vi "Build Xfer Matrix.vi"(7 "NumBins":i32, 8 "error in (no error)":errorcluster, 10 "Voltage":dbl[](array[numeric]), 11 "DMA in":refnum<class "DMA.lvclass">) -> (0 "error out":errorcluster, 2 "xfer":dbl[][](array[numeric]), 3 "DMA out":refnum<class "DMA.lvclass">)   [LabVIEW 2015, in "DMA.lvclass"]
uses:
  DMA.lvclass
  DMA.lvclass/DMA.ctl
  Particle Class/Particle Properties.lvclass/Particle Properties.ctl
  Accessors/Read Particle.vi
  Accessors/Read ri.vi
  Accessors/Read ro.vi
  Accessors/Read Leff.vi
  Accessors/Read Qex.vi
  Accessors/Read Qsh.vi
  Particle Class/Accessors/Write D.vi
  Particle Class/Accessors/Write # of charges.vi
  Particle Class/Calculate Charging Efficiency.vi
  Particle Class/Particle Properties.lvclass
panel:
  out "XY Graph":cluster{dbl[], dbl[]}(graph)
  out "Array 4":dbl[](array[numeric])
  out "kappa":dbl[][][](array[numeric])
  out "Array 2":dbl[][][](array[numeric])
  out "Array":dbl[][][](array[numeric])
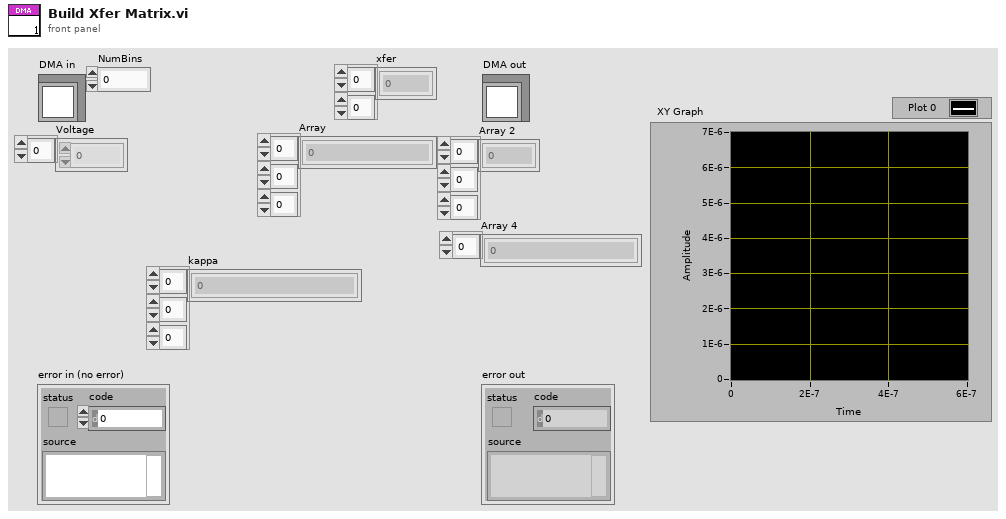
[diagram p1: front panel]
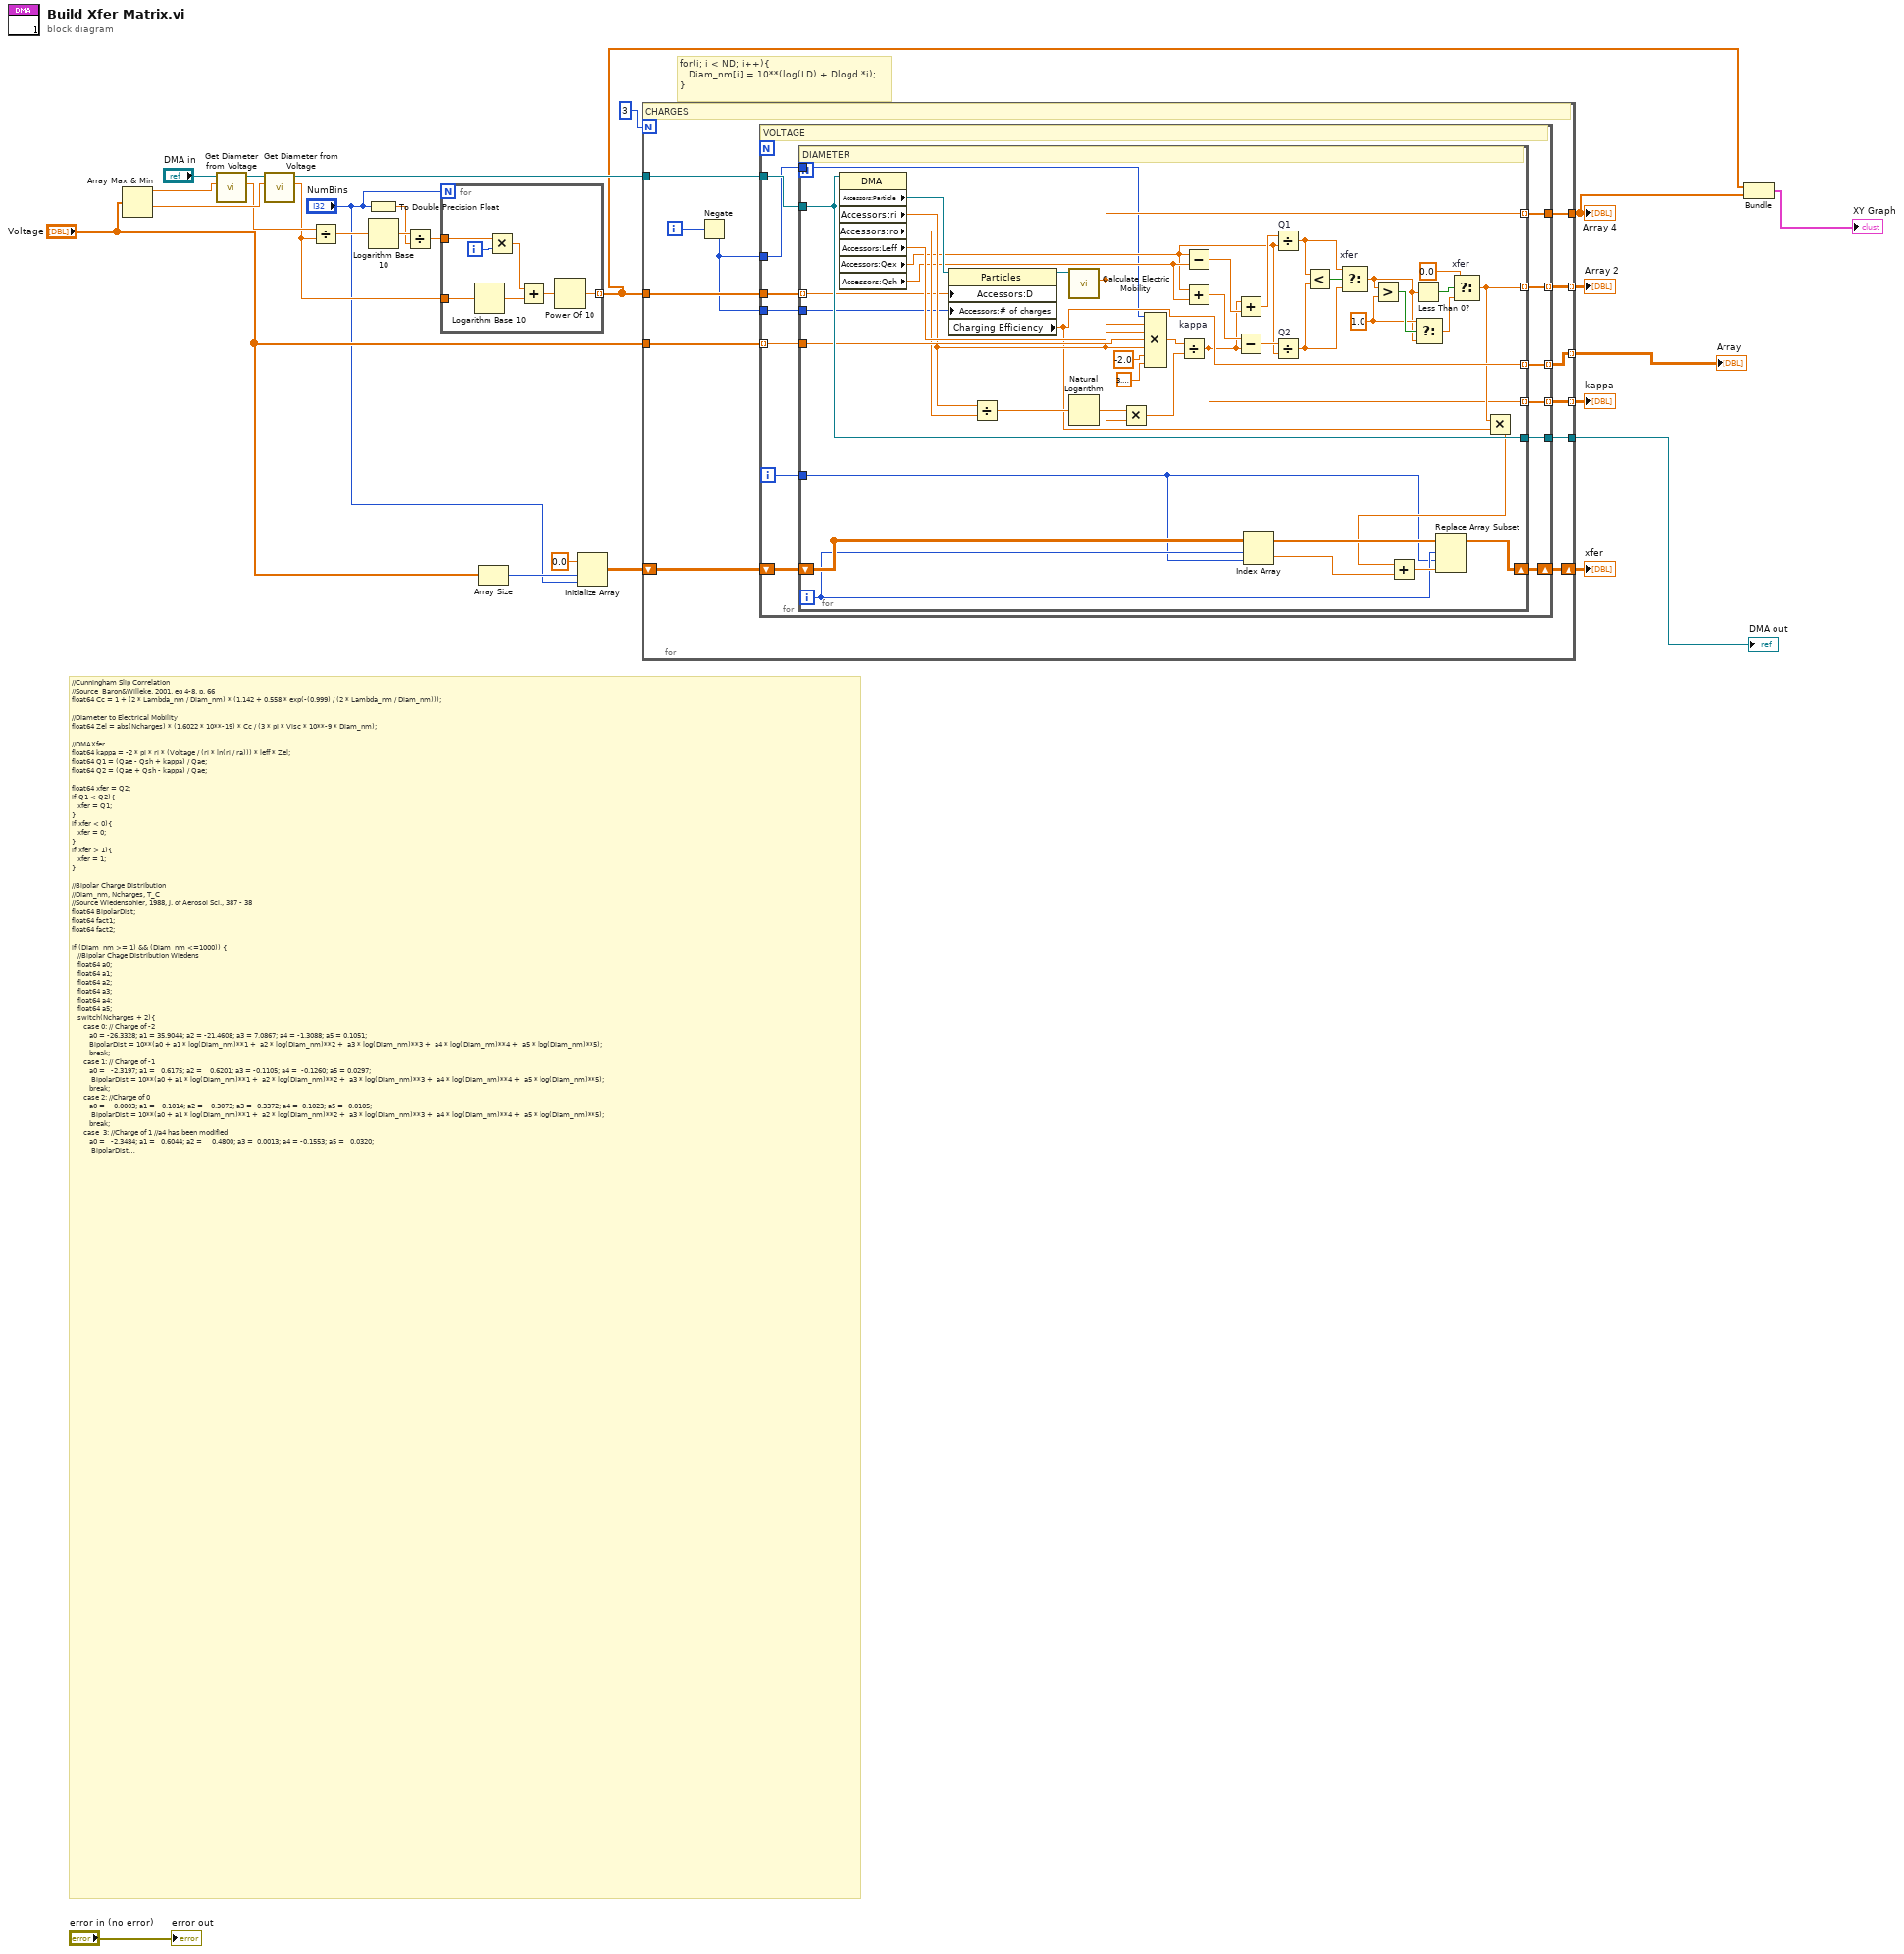
[diagram p0: block diagram]
diagram:
  # "for(i; i < ND; i++){\n   Diam_nm[i] = 10**(log(LD) + Dlogd *i);\n}"
  # "//Cunningham Slip Correlation\n//Source  Baron&Willeke, 2001, eq 4-8, p. 66\nfloat64 Cc = 1 + (2 * Lambda_nm / Diam_nm) * (1.142 + 0.558 * exp(-(0.999) / (2 * Lambda_nm / Diam_nm)));\n\n//Diameter to Electrical Mobility\nfloat64 Zel = abs(Ncharges) * (1.6022 * 10**-19) * Cc / (3 * pi * Visc * 10**-9 * Diam_nm);\n\n//DMAXfer\nfloat64 kappa = -2 * pi * ri * (Voltage / (ri * ln(ri / ra))) * leff * Zel;\nfloat64 Q1 = (Qae - Qsh + kappa) / Qae;\nfloat64 Q2 = (Qae + Qsh - kappa) / Qae;\n\nfloat64 xfer = Q2;\nif(Q1 < Q2){\n   xfer = Q1;\n}\nif(xfer < 0){\n   xfer = 0;\n}\nif(xfer > 1){\n   xfer = 1;\n}\n\n//Bipolar Charge Distribution\n//Diam_nm, Ncharges, T_C\n//Source Wiedensohler, 1988, J. of Aerosol Sci., 387 - 38\nfloat64 BipolarDist;\nfloat64 fact1;\nfloat64 fact2;\n\nif((Diam_nm >= 1) && (Diam_nm <=1000)) {\n   //Bipolar Chage Distribution Wiedens\n   float64 a0;\n   float64 a1;\n   float64 a2;\n   float64 a3;\n   float64 a4;\n   float64 a5;\n   switch(Ncharges + 2){\n      case 0: // Charge of -2\n         a0 = -26.3328; a1 = 35.9044; a2 = -21.4608; a3 = 7.0867; a4 = -1.3088; a5 = 0.1051;\n         BipolarDist = 10**(a0 + a1 * log(Diam_nm)**1 +  a2 * log(Diam_nm)**2 +  a3 * log(Diam_nm)**3 +  a4 * log(Diam_nm)**4 +  a5 * log(Diam_nm)**5);\n         break;\n      case 1: // Charge of -1\n         a0 =   -2.3197; a1 =   0.6175; a2 =    0.6201; a3 = -0.1105; a4 =  -0.1260; a5 = 0.0297;\n          BipolarDist = 10**(a0 + a1 * log(Diam_nm)**1 +  a2 * log(Diam_nm)**2 +  a3 * log(Diam_nm)**3 +  a4 * log(Diam_nm)**4 +  a5 * log(Diam_nm)**5);\n         break;\n      case 2: //Charge of 0\n         a0 =   -0.0003; a1 =  -0.1014; a2 =    0.3073; a3 = -0.3372; a4 =  0.1023; a5 = -0.0105;\n          BipolarDist = 10**(a0 + a1 * log(Diam_nm)**1 +  a2 * log(Diam_nm)**2 +  a3 * log(Diam_nm)**3 +  a4 * log(Diam_nm)**4 +  a5 * log(Diam_nm)**5);\n         break;\n      case  3: //Charge of 1 //a4 has been modified\n         a0 =   -2.3484; a1 =   0.6044; a2 =     0.4800; a3 =  0.0013; a4 = -0.1553; a5 =   0.0320;\n          BipolarDist = 10**(a0 + a1 * log(Diam_nm)**1 +  a2 * log(Diam_nm)**2 +  a3 * log(Diam_nm)**3 +  a4 * log(Diam_nm)**4 +  a5 * log(Diam_nm)**5);\n         break;\n      case  4: //Charge of 2 //a5 has been modified\n         a0 = -44.4756; a1 = 79.3772; a2 =  -62.8900; a3 = 26.4492; a4 = -5.7480; a5 =  0.5049;\n         BipolarDist = 10**(a0 + a1 * log(Diam_nm)**1 +  a2 * log(Diam_nm)**2 +  a3 * log(Diam_nm)**3 +  a4 * log(Diam_nm)**4 +  a5 * log(Diam_nm)**5);\n         break;\n      default:\n         //Bipolar Chage Distribution Gunn\n         fact1 = (1.6022*10**-19) / sqrt(4 * pi**2 * (8.8542*10**-12) * Diam_nm  * 10**-9 * (1.3807*10**-23) * T_K);\n         fact2 = 2 * pi * (8.8542*10**-12) * Diam_nm * 10**-9 * (1.3807*10**-23) * T_K / (1.6022*10**-19) /  (1.6022*10**-19);\n         BipolarDist = fact1 * exp(-1 * (Ncharges - fact2 * ln(1 * 0.875))**2 / 2 / fact2);\n         break;\n   }\n}\nelse {\n   if((Diam_nm > 1000) && (Diam_nm <= 2000)) {\n      //Bipolar Chage Distribution Gunn\n      fact1 = (1.6022*10**-19) / sqrt(4 * pi**2 * (8.8542*10**-12) * Diam_nm  * 10**-9 * (1.3807*10**-23) * T_K);\n      fact2 = 2 * pi * (8.8542*10**-12) * Diam_nm * 10**-9 * (1.3807*10**-23) * T_K / (1.6022*10**-19) /  (1.6022*10**-19);\n      BipolarDist = fact1 * exp(-1 * (Ncharges - fact2 * ln(1 * 0.875))**2 / 2 / fact2);\n   }\n   else{\n      //Return NaN\n      BipolarDist = NaN;\n   }\n}\n\n Output = xfer * BipolarDist;"
  n1 = Array Max & Min(array="Voltage") -> (max value=w24:dbl, min value=w21:dbl)  [unwired: 2 out]
  n2 = call "Get Diameter from Voltage.vi"("Vin"=w24, "DMA in"="DMA in") -> ("Dout"=w19:dbl, "DMA out"=w22:refnum<class "DMA.lvclass">)  [unwired: 7 in, 1 out]
  n3 = call "Get Diameter from Voltage.vi"("Vin"=w21, "DMA in"=w22) -> ("Dout"=w14:dbl, "DMA out"=w20:refnum<class "DMA.lvclass">)  [unwired: 7 in, 1 out]
  n4 = Divide(x=w19, y=w14) -> (x/y=w18:dbl)
  n5 = To Double Precision Float(number="NumBins") -> (double precision float=w16:dbl)
  n6 = Logarithm Base 10(1:w18) -> (0:w17:dbl)
  n7 = Divide(x=w17, y=w16) -> (x/y=w15:dbl)
  n8 = for {
    N: "NumBins" -> [_]
    tunnel: w15 -> [w30]
    tunnel: w14 -> [w33]
    tunnel: [w27] -> w2 mode=indexing
    i -> [w31]
    n9 = Logarithm Base 10(1:w33) -> (0:w32:dbl)
    n10 = Multiply(x=w30, y=w31) -> (x*y=w29:dbl)
    n11 = Add(x=w29, y=w32) -> (x+y=w28:dbl)
    n12 = Power Of 10(x=w28) -> (10^x=w27:dbl)
  }
  n13 = Array Size(array="Voltage") -> (size(s)=w11:i32)
  n14 = Initialize Array(0.0 ("element"), w11, "NumBins") -> (w10:dbl[][])
  n15 = for {
    N: 3 -> [_]
    tunnel: [w45] -> w25
    tunnel: "Voltage" -> [w44]
    tunnel: w20 -> [w43]
    tunnel: w2 -> [w42]
    shift-right: [w40] -> w7
    shift-left: w10 -> [w41]
    tunnel: [w39] -> w6 mode=indexing
    tunnel: [w38] -> w5 mode=indexing
    tunnel: [w37] -> w4 mode=indexing
    tunnel: [w36] -> w3
    i -> [w35]
    # "CHARGES"
    n16 = Negate(x=w35) -> (-x=w34:i32)
    n17 = for {
      tunnel: [w58] -> w45
      tunnel: w44 -> [w57] mode=indexing
      tunnel: w43 -> [w56]
      tunnel: w42 -> [w55]
      tunnel: w34 -> [w54]
      shift-right: [w52] -> w40
      shift-left: w41 -> [w53]
      tunnel: [w50] -> w39 mode=indexing
      tunnel: [w49] -> w38 mode=indexing
      tunnel: [w48] -> w37 mode=indexing
      tunnel: [w47] -> w36
      tunnel: w34 -> [w46]
      i -> [w51]
      # "VOLTAGE"
      n18 = for {
        tunnel: w56 -> [w100]
        tunnel: w57 -> [w95]
        tunnel: [w100] -> w58
        tunnel: w55 -> [w73] mode=indexing
        tunnel: w54 -> [w61]
        shift-right: [w69] -> w52
        shift-left: w53 -> [w70]
        tunnel: w51 -> [w66]
        tunnel: [w64] -> w50 mode=indexing
        tunnel: [w63] -> w49 mode=indexing
        tunnel: [w62] -> w48 mode=indexing
        tunnel: [w60] -> w47 mode=indexing
        tunnel: w46 -> [w59]
        i -> [w67]
        w76 = 1.0 ("y")
        # "DIAMETER"
        n19 = property class="DMA"(reference=w100) -> ("Accessors:Particle"=w99:refnum<class "Particle Properties.lvclass">, "Accessors:ri"=w90:dbl, "Accessors:ro"=w93:dbl, "Accessors:Leff"=w94:dbl, "Accessors:Qex"=w82:dbl, "Accessors:Qsh"=w86:dbl)  [unwired: 1 in, 2 out]
        n20 = property class="Particles"(reference=w99, "Accessors:D"=w73, "Accessors:# of charges"=w61) -> (reference out=w98:refnum<class "Particle Properties.lvclass">, "Charging Efficiency"=w64:dbl)  [unwired: 1 in, 1 out]
        n21 = Divide(x=w90, y=w93) -> (x/y=w92:dbl)
        n22 = call "Calculate Electric Mobility.vi"("Particles in"=w98) -> ("Z"=w60:dbl)  [unwired: 8 in, 2 out]
        n23 = Natural Logarithm(1:w92) -> (0:w91:dbl)
        n24 = Multiply(x=w91, y=w90) -> (x*y=w88:dbl)
        n25 = Compound Arithmetic op=MULTIPLY(w59, w60, w94, w95, w90, -2.0, 3.141592653589793) -> (w89:dbl)
        n26 = Divide "kappa"(x=w89, y=w88) -> (x/y=w62:dbl)
        n27 = Subtract(x=w82, y=w86) -> (x-y=w87:dbl)
        n28 = Add(x=w82, y=w86) -> (x+y=w84:dbl)
        n29 = Add(x=w62, y=w87) -> (x+y=w85:dbl)
        n30 = Subtract(x=w84, y=w62) -> (x-y=w83:dbl)
        n31 = Index Array(array=w70, index (row)=w67, index (col)=w66) -> (element=w72:dbl)
        n32 = Divide "Q1"(x=w85, y=w82) -> (x/y=w80:dbl)
        n33 = Divide "Q2"(x=w83, y=w82) -> (x/y=w79:dbl)
        n34 = Less?(x=w80, y=w79) -> (x < y?=w81:bool)
        n35 = Select "xfer"(t=w80, s=w81, f=w79) -> (s? t:f=w75:dbl)
        n36 = Greater?(x=w75, y=w76) -> (0:w77:bool)
        n37 = Less Than 0?(x=w75) -> (x < 0?=w78:bool)
        n38 = Select(t=w76, s=w77, f=w75) -> (s? t:f=w74:dbl)
        n39 = Select "xfer"(t=0.0, s=w78, f=w74) -> (s? t:f=w63:dbl)
        n40 = Multiply(x=w63, y=w64) -> (x*y=w68:dbl)
        n41 = Add(x=w68, y=w72) -> (x+y=w71:dbl)
        n42 = Replace Array Subset(array=w70, new element=w71, index (row)=w67, index (col)=w66) -> (w69:dbl[][])
      }
    }
  }
  "DMA out" <- w25
  "xfer" <- w7
  "Array" <- w6
  "Array 2" <- w5
  "kappa" <- w4
  "Array 4" <- w3
  n43 = Bundle(w2, w3) -> (→"XY Graph":cluster{dbl[], dbl[]})  [unwired: 1 in]
  "error out" <- "error in (no error)"
